vi "WebService_Startup.vi"(6 "LabVIEW Web Service":refnum<class "Web Service.lvclass">) -> ()   [LabVIEW 2018]
doc: "This VI is just to transmit WebService Status"
uses:
  <vilib>/wsapi/Web Service.lvclass
  GLB_WebService_Status.vi
panel:
  # "Use the web service input terminal to call the VIs on the Service subpalette of the Web Services palette. Do not remove it from the connector pane unless you don't need access to the palette."
  # "Any additional terminals added to the connector pane of a startup VI will be ignored."
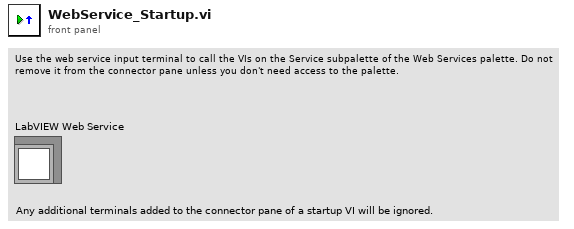
[diagram p1: front panel]
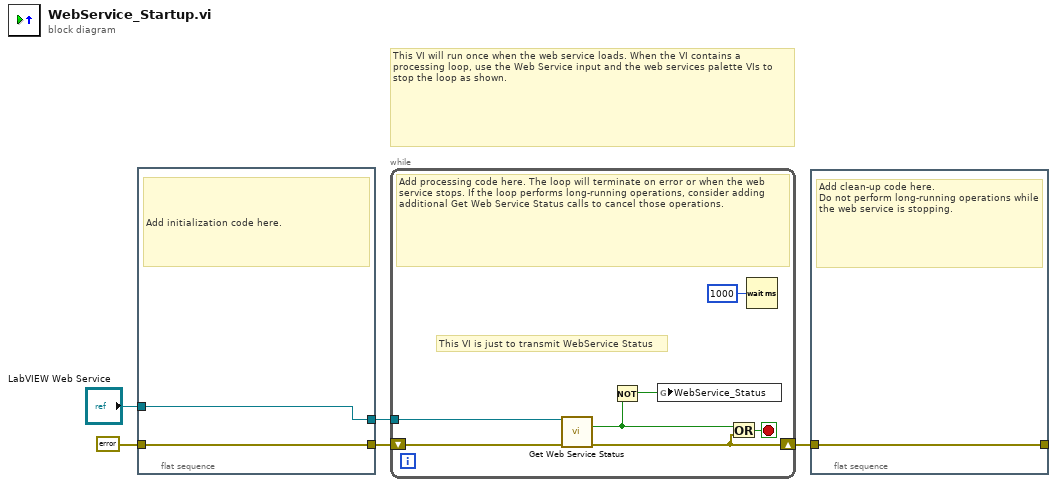
[diagram p0: block diagram]
diagram:
  # "This VI will run once when the web service loads. When the VI contains a processing loop, use the Web Service input and the web services palette VIs to stop the loop as shown."
  n1 = flat-sequence {
    tunnel: "LabVIEW Web Service" -> [w7]
    tunnel: [w7] -> w4
    tunnel: [w6] -> w3
    tunnel: errorcluster {"status"=FALSE, "code"=0, "source"=""} ("error constant") -> [w6]
    frame #0 {
      # "Add initialization code here."
    }
  }
  n2 = while {
    tunnel: w4 -> [w14]
    shift-right: [w11] -> w1
    shift-left: w3 -> [w12]
    stop <- w13 stop-if-true
    # "This VI is just to transmit WebService Status"
    # "Add processing code here. The loop will terminate on error or when the web service stops. If the loop performs long-running operations, consider adding additional Get Web Service Status calls to cancel those operations."
    n3 = call <vilib>:"Get Web Service Status.vi"("LabVIEW Web Service"=w14, "error in (no error)"=w12) -> ("service stopping?"=w9:bool, "error out"=w11:errorcluster)  [unwired: 11 in, 1 out]
    n4 = Not(x=w9) -> (.not. x?=w8:bool)
    n5 = global write "GLB_WebService_Status.vi" "WebService_Status"(w8) -> ()
    n6 = Or(x=w9, y=w11) -> (x .or. y?=w13:bool)
    n7 = Wait (ms)(milliseconds to wait=u32 1000) -> ()  [unwired: 1 out]
  }
  n8 = flat-sequence {
    tunnel: [w15] -> _
    tunnel: w1 -> [w15]
    frame #0 {
      # "Add clean-up code here.\nDo not perform long-running operations while the web service is stopping."
    }
  }
